vi "RSZVB Select More Ratios With Detector.vi"(0 "VISA session":refnum<visa-resource-name>, 1 "Numerator Port Number (1)":i32=1, 2 "Denominator Port Number (1)":i32=1, 3 "Detector (0: RMS)":i32(ring) items=["RMS", "Peak", "Average"], 5 "Channel (1)":i32=1, 7 "Trace Name (Trc1)":string="Trc1", 9 "Source Port (1: Port 1)":i32=1, 11 "error in (no error)":errorcluster {"code" format="%.0x"}, 12 "Denominator Type (0: a)":i32(ring) items=["a", "b"], 13 "Numerator Type (0: a)":i32(ring) items=["a", "b"], 14 "Observation Time (0.01)":dbl=0.01 format="%.2f") -> (4 "dup VISA session":refnum<visa-resource-name>, 15 "error out":errorcluster {"code" format="%.0x"})   [LabVIEW 2011]
doc: "This VI select arbitrary ratios of wave quantities with detector, e.g. for different detectors and source ports or more than 2 ports.\n\nAssigns a measurement parameter to an existing trace or creates a trace and assigns a channel number, a name and a measurement parameter to it. The trace is not displayed.\n\nThe notation for ratios and the VIality of the More Ratios dialog is analogous to the definition of S-parameters.\n\nRatio of wave quantities with port numbers and source port numbers (D<no> for drive port; the source port for the numerator and the denominator can be equal or different).\n\nRemote-control command(s):\nCALCulate<Ch>:PARameter:SDEFine '<string>', 'B2D1/A1D1SAM' | 'B1D1/A1D1RMS' | 'B2D1/B1D1PEAK' | 'B1D1/B2D1SAM' | ...\nCALCulate<Ch>:PARameter:MEASure '<string>', 'B2D1/A1D1SAM' | 'B1D1/A1D1RMS' | 'B2D1/B1D1PEAK' | 'B1D1/B2D1SAM' | ...\n[SENSe<Ch>:]SWEep:DETector:TIME"
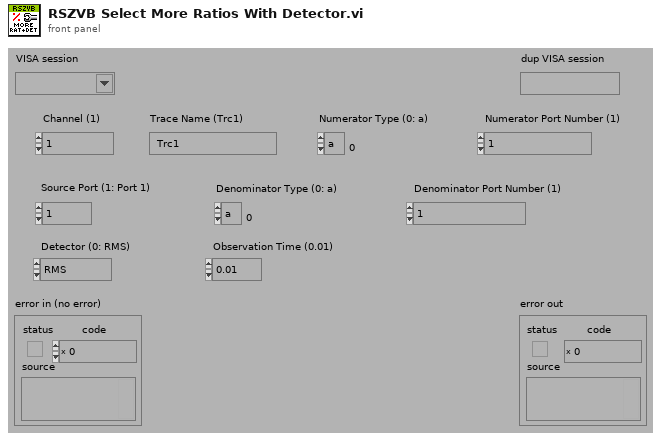
[diagram p1: front panel]
types:
  T1 = cluster{"Error Checking (T: On)":bool, "Installed Options":string[], "Data Valid?":bool, "Ports":i32, "Model":string[], "Option Checking (T: On)":bool}
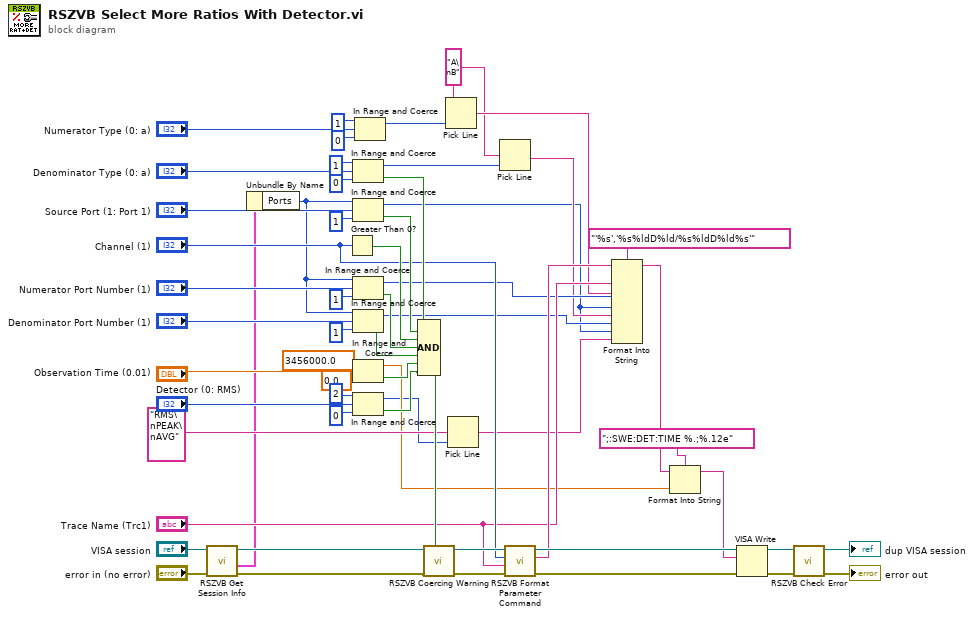
[diagram p0: block diagram]
diagram:
  w26 = "A\nB"
  n1 = call "RSZVB Get Session Info.vi"("error in (no error)"="error in (no error)", "VISA session"="VISA session") -> ("error out"=w4:errorcluster, "Session Info"=w2:T1, "dup VISA session"=w3:refnum<visa-resource-name>)  [unwired: 7 in]
  n2 = Unbundle By Name(w2) -> ("Ports"=w1:i32)
  n3 = Greater Than 0?(x="Channel (1)") -> (x > 0?=w42:bool)
  n4 = In Range and Coerce(upper limit=1, x="Denominator Type (0: a)", lower limit=0) -> (coerced(x)=w45:i32, In Range?=w44:bool)
  n5 = In Range and Coerce(upper limit=w1, x="Source Port (1: Port 1)", lower limit=1) -> (coerced(x)=w23:i32, In Range?=w43:bool)
  n6 = In Range and Coerce(upper limit=w1, x="Numerator Port Number (1)", lower limit=1) -> (coerced(x)=w28:i32, In Range?=w41:bool)
  n7 = In Range and Coerce(upper limit=w1, x="Denominator Port Number (1)", lower limit=1) -> (coerced(x)=w25:i32, In Range?=w40:bool)
  n8 = In Range and Coerce(upper limit=3456000.0, x="Observation Time (0.01)", lower limit=0.0) -> (coerced(x)=w10:dbl, In Range?=w16:bool)
  n9 = In Range and Coerce(upper limit=2, x="Detector (0: RMS)", lower limit=0) -> (coerced(x)=w8:i32, In Range?=w20:bool)
  n10 = In Range and Coerce(upper limit=1, x="Numerator Type (0: a)", lower limit=0) -> (coerced(x)=w29:i32)  [unwired: 1 out]
  n11 = Compound Arithmetic op=AND(w44, w43, w42, w41, w40, w16, w20) -> (w55:bool)
  n12 = call "RSZVB Coercing Warning.vi"("In Range?"=w55, "error in (no error)"=w4, "VISA session"=w3) -> ("error out"=w53:errorcluster, "dup VISA session"=w52:refnum<visa-resource-name>)  [unwired: 7 in]
  n13 = Pick Line(multi-line string=w26, line index=w29) -> (output string=w27:string)  [unwired: 1 in]
  n14 = Pick Line(multi-line string="RMS\nPEAK\nAVG", line index=w8) -> (output string=w13:string)  [unwired: 1 in]
  n15 = Pick Line(multi-line string=w26, line index=w45) -> (output string=w24:string)  [unwired: 1 in]
  n16 = call "RSZVB Format Parameter Command.vi"("error in (no error)"=w53, "Trace Name (Trc1)"="Trace Name (Trc1)", "Channel (1)"="Channel (1)", "VISA session"=w52) -> ("error out"=w54:errorcluster, "Buffer"=w49:string, "dup VISA session"=w51:refnum<visa-resource-name>)  [unwired: 5 in]
  n17 = Format Into String(format string="'%s','%s%ldD%ld/%s%ldD%ld%s'", initial string=w49, "Trace Name (Trc1)", w27, w28, w23, w24, w25, w23, w13) -> (resulting string=w12:string)  [unwired: 1 in, 1 out]
  n18 = Format Into String(format string=";:SWE:DET:TIME %.;%.12e", initial string=w12, w10) -> (resulting string=w11:string)  [unwired: 1 in, 1 out]
  n19 = VISA Write(VISA resource name=w51, write buffer=w11, error in (no error)=w54) -> (VISA resource name out=w56:refnum<visa-resource-name>, error out=w57:errorcluster)  [unwired: 1 out]
  n20 = call "RSZVB Check Error.vi"("error in (no error)"=w57, "VISA session"=w56) -> ("error out"=→"error out":errorcluster, "dup VISA session"=→"dup VISA session":refnum<visa-resource-name>)  [unwired: 8 in]
